vi "Set Item Data.vi"(8 "error in (no error)":errorcluster, 10 "Front Panel Controls":T1, 11 "Item in":refnum<class "Item.lvclass">) -> (0 "error out":errorcluster, 3 "Item out":refnum<class "Item.lvclass">)   [LabVIEW 2020, in "VI Properties Editor.lvlib" / "Item.lvclass"]
doc: "Sets the values of <B>Front Panel Controls</B> to the values of the data of <B>Item in</B>."
uses:
  Item.lvclass
  CTLs/Main Front Panel Controls.ctl
  VI Properties Editor.lvlib
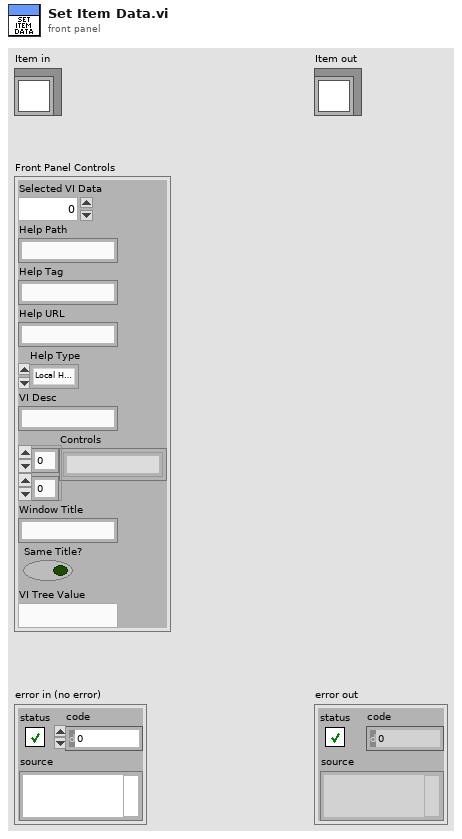
[diagram p1: front panel]
types:
  T1 = typedef "VI Properties Editor.lvlib/Main Front Panel Controls.ctl" = cluster{"Selected VI Data":i32, "Help Path":string, "Help Tag":string, "Help URL":string, "Help Type":enum16{"Local Help File", "Web-based Help"}, "VI Desc":string, "Controls":string[][], "Window Title":string, "Same Title?":bool, "VI Tree Value":string}
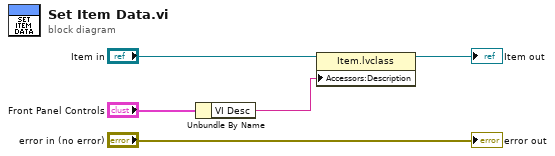
[diagram p0: block diagram]
diagram:
  n1 = Unbundle By Name("Front Panel Controls") -> ("VI Desc"=w2:string)
  n2 = property class="Item.lvclass"(reference="Item in", "Accessors:Description"=w2) -> (reference out=→"Item out":refnum<class "Item.lvclass">)  [unwired: 1 in, 1 out]
  "error out" <- "error in (no error)"
